vi "Create Header String.vi"(5 "File Name":string, 6 "File Format":T1(ring), 8 "User Comments":string="This data's for you!\nType \u0011-H to get a help window for the various controls.", 11 "File Info Input":T5={"FilePath"=path "/DATA/Labview Items", "Field (T)"=55.0, "Temperature (K)"=77.0, "X-Axis"=enum."nm", "Center nm"=55.0, "Current Grating Density"=enum."600", "CCD Parameters"={"Exposure Time (s)"=0.2, "Offset"=0.0, "BkgrdCrct"=FALSE, "Shutter"=FALSE, "Mode"=enum."Regular", "Repetition"=4, "dt or s"=0.0}, "Operation Mode"=enum."NML Data Acquisition", "Exp Index"=0, "Index_repetition"=0, "Index"=0, "Current Detector"=enum."CCD-1024x256"} {"CCD Parameters"."dt or s" format="%#.6f"; "CCD Parameters"."Repetition" min=1; "CCD Parameters"."Offset" format="%#.2f"; "CCD Parameters"."Exposure Time (s)" min=0.02 max=6000.0 format="%#.2f"; "Center nm" format="%.2f"; "Temperature (K)" format="%.2f"; "Field (T)" format="%.2f"}) -> (0 "Contents Written":string)   [LabVIEW 2019]
uses:
  Globals and TypeDefs/Type Definitions.llb/FileInfoParameter.ctt
  Globals and TypeDefs/Type Definitions.llb/Wavelength Unit.ctt
  Globals and TypeDefs/Type Definitions.llb/McPherson Grating Density.ctl
  Globals and TypeDefs/Type Definitions.llb/CCDParameter.ctt
  Globals and TypeDefs/Type Definitions.llb/OperationMode.ctt
  Globals and TypeDefs/Type Definitions.llb/ListOfDetectors.ctt
  File and save/X-Axis Converter.llb/X-Point Converter.vi
panel:
  out "Current Detector":T2
  out "Operation Mode":T3
  out "Current Grating Density":enum16{"150", "300", "600", "1200", "1800"}(ring)
  in  "Header Item":T4(ring)=enum."Experiment Index & Time Stamp"
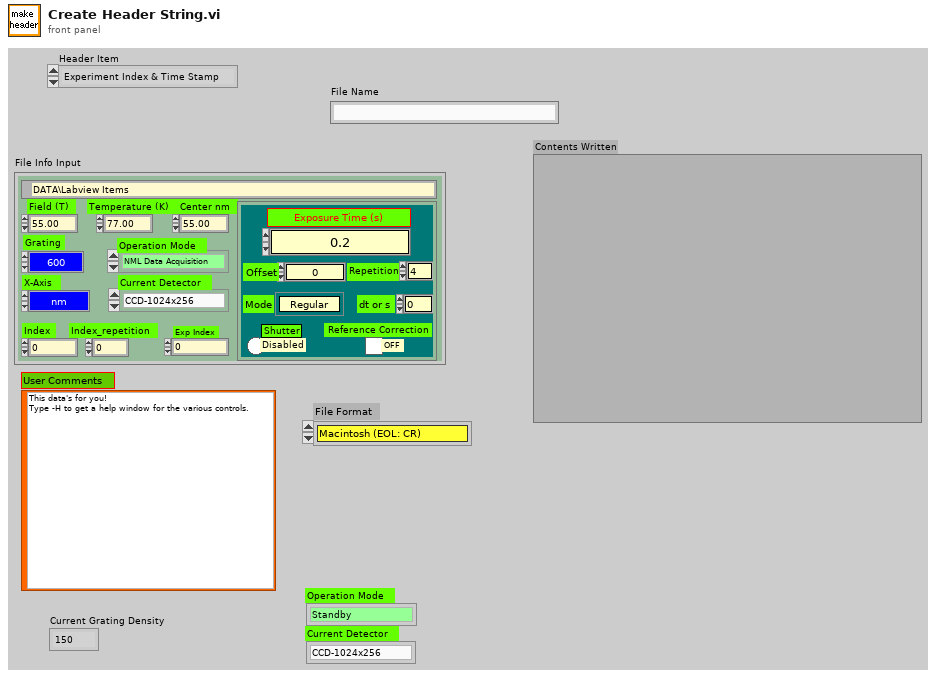
[diagram p1: front panel]
types:
  T1 = enum16{"Macintosh (EOL: CR)", "Unix (EOL: LF)", "DOS/Windows (EOL: CR+LF)"}
  T2 = typedef "ListOfDetectors.ctt" = enum8{"CCD-1024x256", "InGaAs PDA-1024x1", "CCD-1340x400", "Ge Single Channel", "Si Single Channel", "PMT Single Channel"}
  T3 = typedef "OperationMode.ctt" = enum16{"Standby", "CCD Single Shot", "CCD Sequence Shots", "CCD Custom Shots", "CCD Reference Shot", "Step Scanning ", "Time Scanning", "NML Data Acquisition"}
  T4 = enum16{"--Quit--", "Experiment Index & Time Stamp", "File Path", "Center Wavelength", "Temperature", "Field & Magnet ID", "Operation Mode & Detector", "Exposure Time & Offset", "User Comments", "Misc"}
  T5 = typedef "FileInfoParameter.ctt" = cluster{"FilePath":path, "Field (T)":dbl, "Temperature (K)":dbl, "X-Axis":T6, "Center nm":dbl, "Current Grating Density":T7, "CCD Parameters":T8, "Operation Mode":T3, "Exp Index":u32, "Index_repetition":u16, "Index":u16, "Current Detector":T2}
  T6 = typedef "Wavelength Unit.ctt" = enum8{"Point", "nm", "eV", "meV", "cm_1"}
  T7 = typedef "McPherson Grating Density.ctl" = enum8{"150", "300", "600", "1200", "1800"}
  T8 = typedef "CCDParameter.ctt" = cluster{"Exposure Time (s)":dbl, "Offset":dbl, "BkgrdCrct":bool, "Shutter":bool, "Mode":enum8{"Regular", "OverExp Cor", "SpikeRemove", "ForCalibration"}, "Repetition":u16, "dt or s":dbl}
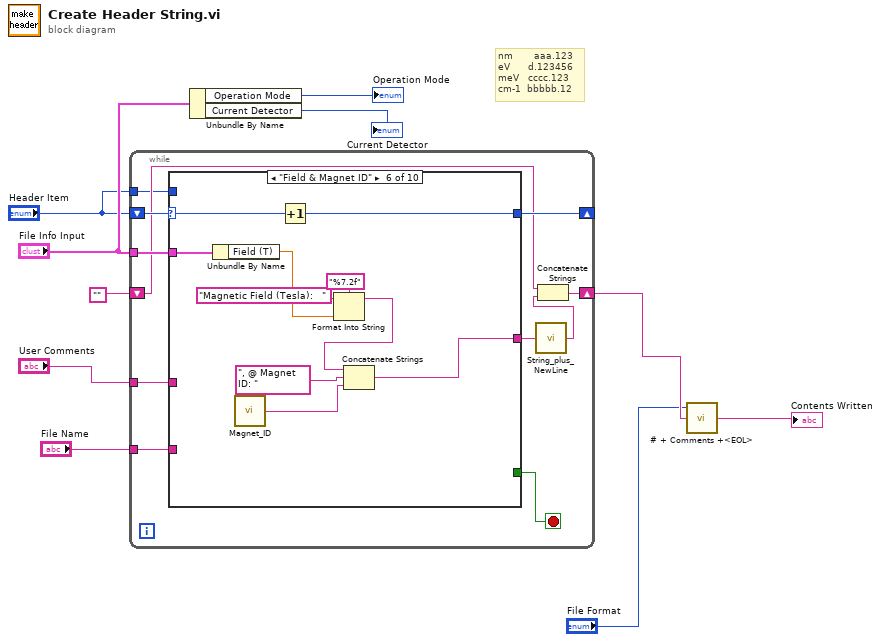
[diagram p0: block diagram]
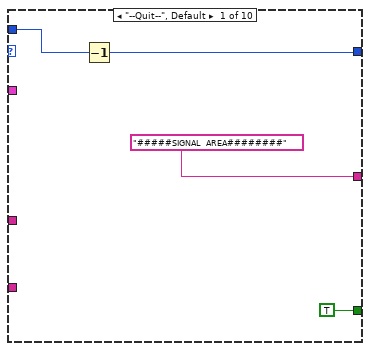
[diagram p2: hidden frame]
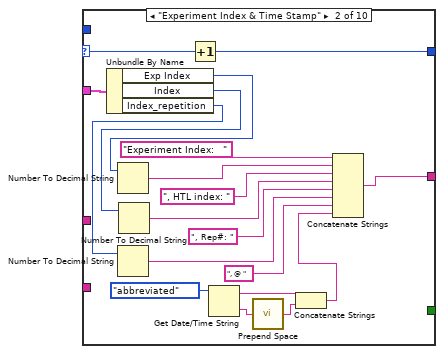
[diagram p3: hidden frame]
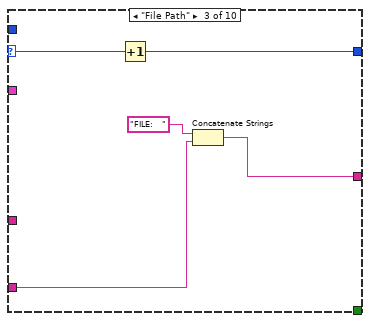
[diagram p4: hidden frame]
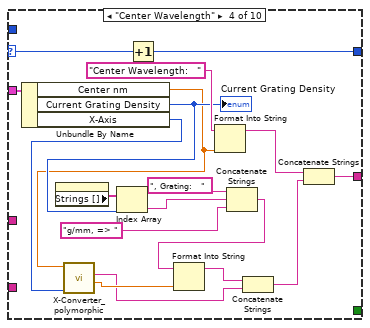
[diagram p5: hidden frame]
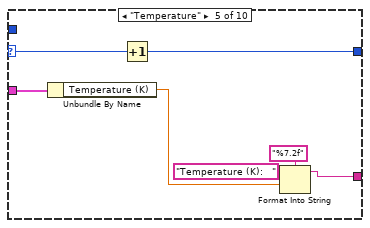
[diagram p6: hidden frame]
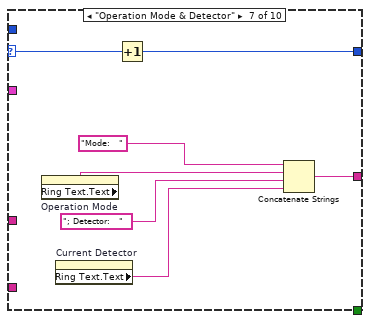
[diagram p7: hidden frame]
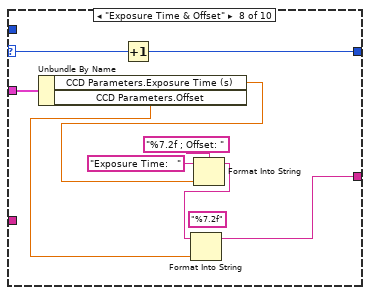
[diagram p8: hidden frame]
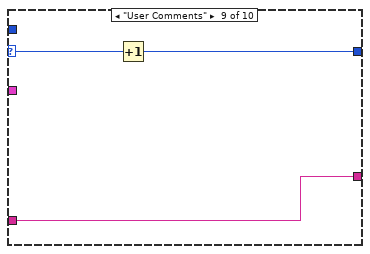
[diagram p9: hidden frame]
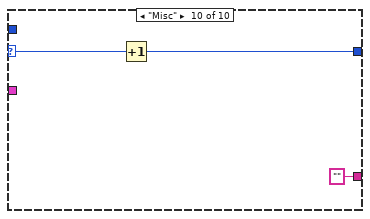
[diagram p10: hidden frame]
diagram:
  # "nm       aaa.123\neV      d.123456\nmeV   cccc.123\ncm-1  bbbbb.12"
  n1 = while {
    shift-right: [w21] -> _
    shift-left: "Header Item" -> [w20]
    tunnel: "File Info Input" -> [w19]
    shift-right: [w18] -> w4
    shift-left: "" -> [w15]
    tunnel: "User Comments" -> [w14]
    tunnel: "File Name" -> [w11]
    tunnel: "Header Item" -> [w12]
    stop <- w13 stop-if-true
    n2 = case shown="\"Field & Magnet ID\"" w20 {
      selector: w20 -> [_ w43 w48 w66 w73 w83 w90 w99 w102 w105]
      tunnel: [w23 w44 w49 w67 w74 w84 w91 w100 w103 w104] -> w21
      tunnel: w19 -> [_ w42 _ w64 w72 w82 _ w98 _ _]
      tunnel: ["#####SIGNAL  AREA########" w36 w45 w50 w68 w75 w85 w92 w101 "" ("User Comments")] -> w16
      tunnel: w14 -> [_ _ _ _ _ _ _ _ w101 _]
      tunnel: w11 -> [_ _ w46 _ _ _ _ _ _ _]
      tunnel: [TRUE _ _ _ _ _ _ _ _ _] -> w13
      tunnel: w12 -> [w24 _ _ _ _ _ _ _ _ _]
      frame "--Quit--", Default {
        n3 = Decrement(x=w24) -> (x-1=w23:T4)
      }
      frame "Experiment Index & Time Stamp" {
        n4 = Unbundle By Name(w42) -> ("Exp Index"=w39:u32, "Index"=w38:u16, "Index_repetition"=w37:u16)
        n5 = Number To Decimal String(number=w39) -> (decimal integer string=w40:string)  [unwired: 1 in]
        n6 = Number To Decimal String(number=w37) -> (decimal integer string=w32:string)  [unwired: 1 in]
        n7 = Number To Decimal String(number=w38) -> (decimal integer string=w34:string)  [unwired: 1 in]
        n8 = Increment(x=w43) -> (x+1=w44:T4)
        n9 = Get Date/Time String(date format (0)=enum16{"short", "long", "abbreviated"}."abbreviated") -> (date string=w30:string, time string=w27:string)  [unwired: 2 in]
        n10 = call "Prepend Space.vi"("Input String"=w27) -> ("Space + Input String"=w26:string)
        n11 = Concatenate Strings(w30, w26) -> (w28:string)
        n12 = Concatenate Strings("Experiment Index:   " ("string"), w40, ", HTL index: " ("string"), w34, ", Rep#: " ("string"), w32, ", @ " ("string"), w28) -> (w36:string)
      }
      frame "File Path" {
        n13 = Increment(x=w48) -> (x+1=w49:T4)
        n14 = Concatenate Strings("FILE:   ", w46) -> (w45:string)
      }
      frame "Center Wavelength" {
        n15 = Unbundle By Name(w64) -> ("Center nm"=w56:dbl, "Current Grating Density"=w58:T7, "X-Axis"=w57:T6)
        "Current Grating Density" <- w58
        n16 = property on="Current Grating Density" class="Enum (strict)"() -> ("Strings []"=w59:string[])  [unwired: 2 in, 2 out]
        n17 = call-poly "X-Converter_polymorphic.vi"("X-Axis Unit"=w57, "X-Axis input"=w56) -> ("X-Axis Output"=w54:dbl, "X-Axis Unit String"=w52:string)  [unwired: 3 in, 2 out]
        n18 = Index Array(array=w59, index=w58) -> (element=w61:string)
        n19 = Increment(x=w66) -> (x+1=w67:T4)
        n20 = Format Into String(initial string="Center Wavelength:   ", w56) -> (resulting string=w63:string)  [unwired: 2 in, 1 out]
        n21 = Concatenate Strings(", Grating:   ", w61, "g/mm, => " ("string")) -> (w55:string)
        n22 = Format Into String(initial string=w55, w54) -> (resulting string=w53:string)  [unwired: 2 in, 1 out]
        n23 = Concatenate Strings(w53, w52) -> (w51:string)
        n24 = Concatenate Strings(w63, w51) -> (w50:string)
      }
      frame "Temperature" {
        n25 = Unbundle By Name(w72) -> ("Temperature (K)"=w69:dbl)
        n26 = Increment(x=w73) -> (x+1=w74:T4)
        n27 = Format Into String(format string="%7.2f", initial string="Temperature (K):   ", w69) -> (resulting string=w68:string)  [unwired: 1 in, 1 out]
      }
      frame "Field & Magnet ID" {
        n28 = Unbundle By Name(w82) -> ("Field (T)"=w78:dbl)
        n29 = call "Magnet_ID.VI"() -> ("Cell"=w77:string)
        n30 = Increment(x=w83) -> (x+1=w84:T4)
        n31 = Format Into String(format string="%7.2f", initial string="Magnetic Field (Tesla):   ", w78) -> (resulting string=w76:string)  [unwired: 1 in, 1 out]
        n32 = Concatenate Strings(w76, ", @ Magnet ID: ", w77) -> (w75:string)
      }
      frame "Operation Mode & Detector" {
        n33 = property on="Operation Mode" class="Enum (strict)"() -> ("Ring Text.Text"=w88:string)  [unwired: 2 in, 2 out]
        n34 = property on="Current Detector" class="Enum (strict)"() -> ("Ring Text.Text"=w86:string)  [unwired: 2 in, 2 out]
        n35 = Increment(x=w90) -> (x+1=w91:T4)
        n36 = Concatenate Strings("Mode:   ", w88, "; Detector:   ", w86) -> (w85:string)
      }
      frame "Exposure Time & Offset" {
        (unwired) "%7.2f"
        n37 = Unbundle By Name(w98) -> ("CCD Parameters.Exposure Time (s)"=w95:dbl, "CCD Parameters.Offset"=w93:dbl)
        n38 = Increment(x=w99) -> (x+1=w100:T4)
        n39 = Format Into String(format string="%7.2f ; Offset: ", initial string="Exposure Time:   ", w95) -> (resulting string=w94:string)  [unwired: 1 in, 1 out]
        n40 = Format Into String(initial string=w94, w93) -> (resulting string=w92:string)  [unwired: 2 in, 1 out]
      }
      frame "User Comments" {
        n41 = Increment(x=w102) -> (x+1=w103:T4)
      }
      frame "Misc" {
        n42 = Increment(x=w105) -> (x+1=w104:T4)
      }
    }
    n43 = call "String_plus_NewLine.vi"("Input String"=w16) -> ("Input String +[\\n]"=w17:string)
    n44 = Concatenate Strings(w15, w17) -> (w18:string)
  }
  n45 = Unbundle By Name("File Info Input") -> ("Operation Mode"=→"Operation Mode":T3, "Current Detector"=→"Current Detector":T2)
  n46 = call "# + Comments +<EOL>.vi"("Input String"=w4, "File Format"="File Format") -> ("Output String"=→"Contents Written":string)  [unwired: 1 in]
